vi "ProgressBar.vi"(9 "Bounds":T1, 11 "Settings":T4={"Name of test"="", "Date"=timestamp(0 s since 1904-01-01), "Location"="", "Template"="", "Soundcard"="", "resolution"=32, "Sampling rate"=48000, "Ch1 Gain "=25.0, "Ch2 Gain"=10.0, "Sample time (s)"=0.3, "Pre-trigger (s)"=0.01, "Hammer Threshold"=10.0, "Positions"=12, "Taps/Position"=5, "Set Names"="", "Freq resolution"=10.0, "Hammer cutoff"=0.0, "Mic cutoff"=0.0, "Double bounce "=0.0, "Hammer Cal"=10.0, "dB Offset"=0.0, "Accel Cal"=10.0, "Vibrometer Cal"=0.0, "Mic Cal"=0.0, "Output"=2, "Voltage Cal"=1.0, "Vibrometer Port"="ASRL27::INSTR", "Range"=4, "High Pass"=2, "Bandwidth"=4, "X Range"=[], "Y Range"=[], "dB Spread"=0.0, "Trigger"=0, "Ch_1"=25, "Ch_2"=25, "flip?"=FALSE, "60Hz"=FALSE, "Time offset"=0.0, "Piezo Cal"=1.0, "Default Notes"=""} {"Ch_2" min=1 step=1; "Ch_1" min=1 max=100 step=1; "Trigger" items=["Hammer (force)", "Self-tap", "Spacebar"]; "Bandwidth" items=["1 kHz"=1, "5 kHz"=5, "10 kHz"=10, "25 kHz"=25, "50 kHz"=50, "100 kHz"=100]; "High Pass" items=["Off", "13 Hz", "104 Hz"]; "Range" items=["10 mm/s"=1, "20 mm/s"=2, "50 mm/s"=5, "100 mm/s"=10, "200 mm/s"=20, "500 mm/s"=50, "1 m/s"=100, "2 m/s"=200]; "Output" items=["Accelerometer", "Speed (from acceleration)", "Microphone", "Vibrometer", "Piezo"]; "Voltage Cal" format="%#_13g"; "Ch2 Gain" format="%#_13g"; "Ch1 Gain" format="%#_13g"; "Double bounce" min=0.0; "Mic cutoff" min=0.0 format="%#_4g"; "Hammer cutoff" min=0.0 format="%#_4g"; "Freq resolution" min=0.0; "Pre-trigger (s)" format="%#_13g"; "Date" format="%<%H:%M\n%d/%m/%y>T"; "resolution" items=["16 bit"=16, "24 bit"=24, "32 bit"=32]; "Sampling rate" items=["22050 samp/s"=22050, "44100 samp/s"=44100, "48000 samp/s"=48000]}) -> (1 "files":string[](array[string]), 2 "positions":T2(array[cluster]), 3 "Progress Bar":picture)   [LabVIEW 2022 SP3]
uses:
  PreferencesControl.ctl
  <vilib>/Utility/miscctls.llb/LVBoundsTypeDef.ctl
panel:
  in  "Windows":T3={"Font Name:"="Times", "Size"=18, "Strikeout?"=FALSE, "Italic?"=FALSE, "Underline?"=FALSE, "Outline?"=FALSE, "Shadow?"=FALSE, "Bold?"=FALSE}
  out "Existing Data":string[](array[string])
  in  "Mac":T3={"Font Name:"="Times", "Size"=14, "Strikeout?"=FALSE, "Italic?"=FALSE, "Underline?"=FALSE, "Outline?"=FALSE, "Shadow?"=FALSE, "Bold?"=FALSE}
  # "Hz"
  # "dB"
  # "dB"
  # "sec"
  # "sec"
  # "mV/Pa"
  # "mV/m/s2"
  # "mV/mm/s"
  # "V/N"
  # "sec"
  # "sec"
  # "mV/N"
  # "a.u."
  # "a.u."
  # "sec"
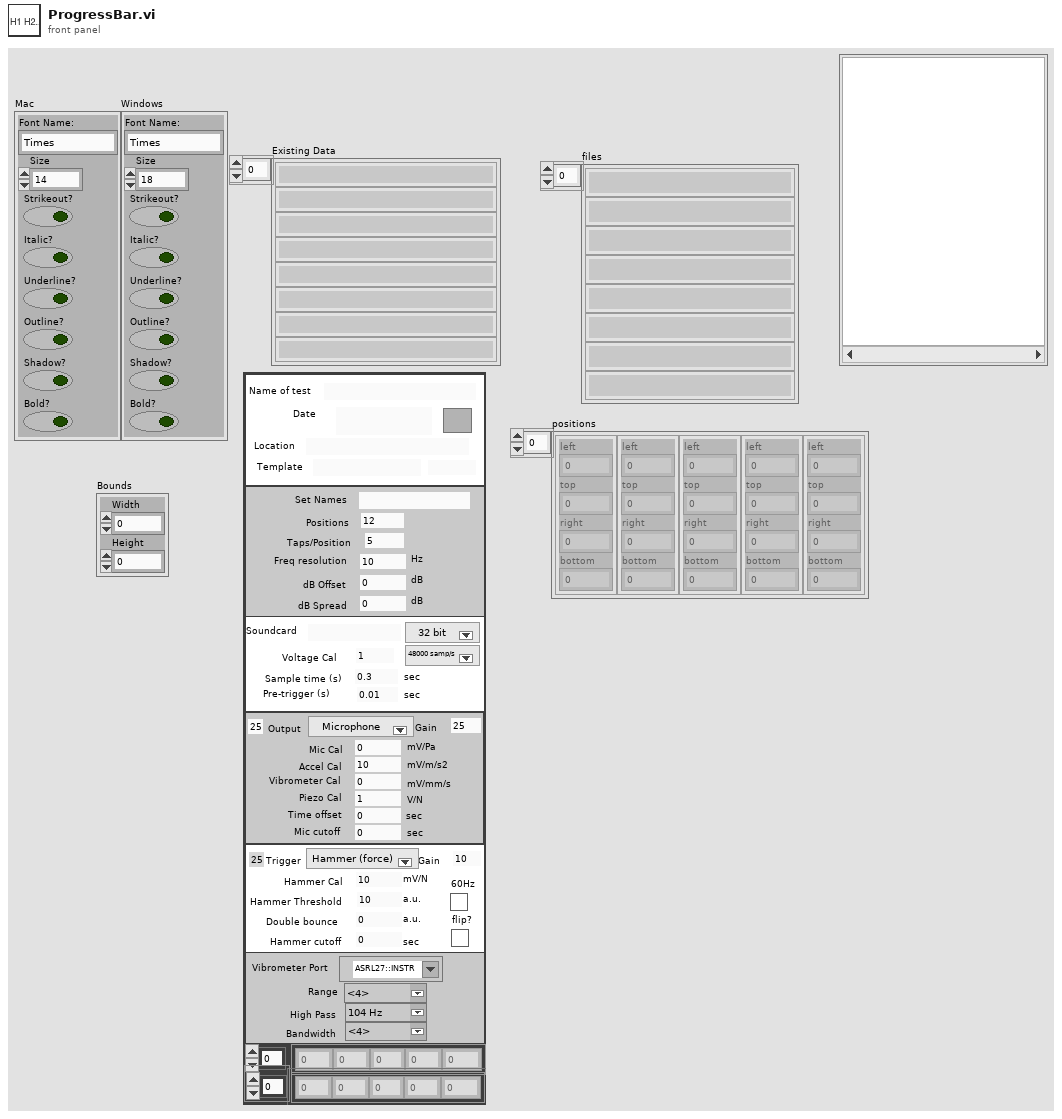
[diagram p1: front panel]
types:
  T1 = typedef "LVBoundsTypeDef.ctl" = cluster{"Width":u32, "Height":u32}
  T2 = cluster{"left":i16, "top":i16, "right":i16, "bottom":i16}[]
  T3 = cluster{"Font Name:":string, "Size":i16, "Strikeout?":bool, "Italic?":bool, "Underline?":bool, "Outline?":bool, "Shadow?":bool, "Bold?":bool}
  T4 = typedef "PreferencesControl.ctl" = cluster{"Name of test":string, "Date":timestamp, "Location":string, "Template":string, "Soundcard":string, "resolution":u16, "Sampling rate":u16, "Ch1 Gain ":dbl, "Ch2 Gain":dbl, "Sample time (s)":dbl, "Pre-trigger (s)":dbl, "Hammer Threshold":dbl, "Positions":i16, "Taps/Position":i16, "Set Names":string, "Freq resolution":dbl, "Hammer cutoff":dbl, "Mic cutoff":dbl, "Double bounce ":dbl, "Hammer Cal":dbl, "dB Offset":dbl, "Accel Cal":dbl, "Vibrometer Cal":dbl, "Mic Cal":dbl, "Output":u16, "Voltage Cal":dbl, "Vibrometer Port":refnum<visa-resource-name>, "Range":u16, "High Pass":u16, "Bandwidth":u16, "X Range":cluster{"Minimum":dbl, "Maximum":dbl, "Increment":dbl, "Minor Increment":dbl, "Start":dbl}[], "Y Range":cluster{"Minimum":dbl, "Maximum":dbl, "Increment":dbl, "Minor Increment":dbl, "Start":dbl}[], "dB Spread":dbl, "Trigger":u16, "Ch_1":u8, "Ch_2":u8, "flip?":bool, "60Hz":bool, "Time offset":dbl, "Piezo Cal":dbl, "Default Notes":string}
  T5 = enum16{"User-specified Font", "Application Font", "System Font", "Dialog Font"}
  T6 = cluster{"Width":i16, "Style":enum32{"Solid", "Dash", "Dot", "DashDot", "DashDotDot"}}
  T7 = cluster{"left":i16, "top":i16, "right":i16, "bottom":i16}
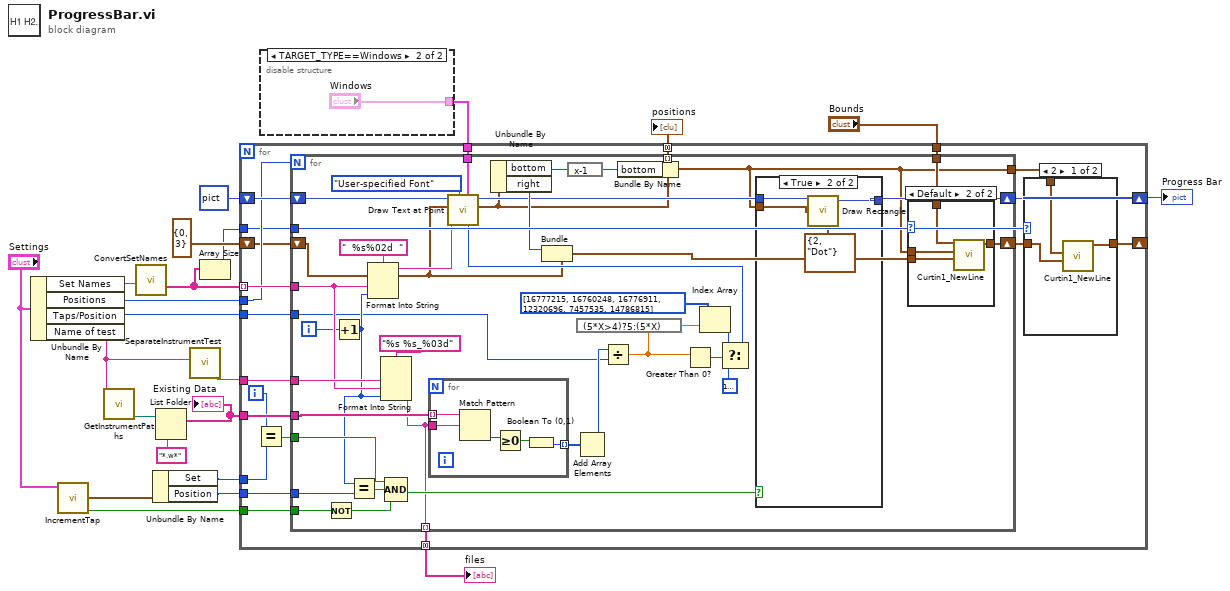
[diagram p0: block diagram]
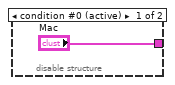
[diagram p2: hidden frame]
diagram:
  n1 = Unbundle By Name("Settings") -> ("Set Names"=w15:string, "Positions"=w14:i16, "Taps/Position"=w13:i16, "Name of test"=w5:string)
  n2 = call "IncrementTap.vi"("Settings"="Settings") -> ("Done?"=w9:bool, "Location"=w12:cluster{"Set":i16, "Position":i16, "Tap":i16})  [unwired: 5 in, 4 out]
  n3 = call "GetInstrumentPaths.vi"("Instrument"=w5) -> ("Path To Raw Folder"=w17:path)  [unwired: 6 in, 4 out]
  n4 = call "ConvertSetNames.vi"("Set Names"=w15) -> ("Set Names"=w2:string[])  [unwired: 10 in]
  n5 = Unbundle By Name(w12) -> ("Set"=w11:i16, "Position"=w10:i16)
  n6 = List Folder(path=w17, pattern="*.w*") -> (filenames=w18:string[])  [unwired: 2 in, 3 out]
  "Existing Data" <- w18
  n7 = call "SeparateInstrumentTest.vi"("Instrument"=w5) -> ("Just test"=w4:string)  [unwired: 6 in, 4 out]
  n8 = Array Size(array=w2) -> (size(s)=w1:i32)
  n9 = disable-structure shown="TARGET_TYPE==Windows" {
    disable-tunnel: ["Mac" "Windows"] -> w19
    frame condition #0 (active) {
    }
    frame condition #1 {
    }
  }
  n10 = for {
    tunnel: w2 -> [w45] mode=indexing
    tunnel: w14 -> [w42]
    shift-right: [w43] -> w21
    shift-left: picture data[5B] ("new picture") -> [w44]
    shift-right: [w27] -> _
    shift-left: cluster{"x":i16, "y":i16} {"x"=0, "y"=3} ("origin") -> [w41]
    tunnel: w19 -> [w40]
    tunnel: w4 -> [w39]
    tunnel: w18 -> [w38]
    tunnel: w13 -> [w37]
    tunnel: w11 -> [w35]
    tunnel: w10 -> [w34]
    tunnel: w9 -> [w32]
    tunnel: [w31] -> w7 mode=concatenating
    tunnel: [w30] -> w6 mode=concatenating
    tunnel: "Bounds" -> [w29]
    tunnel: w1 -> [w28]
    i -> [w36]
    n11 = Equal?(x=w36, y=w35) -> (x = y?=w33:bool)
    n12 = for {
      N: w42 -> [_]
      tunnel: w45 -> [w73]
      shift-right: [w67] -> w43
      shift-left: w44 -> [w88]
      shift-right: [w53] -> w26
      shift-left: w41 -> [w57]
      tunnel: w40 -> [w86]
      tunnel: w39 -> [w83]
      tunnel: w38 -> [w82]
      tunnel: w37 -> [w55]
      tunnel: w34 -> [w71]
      tunnel: w33 -> [w69]
      tunnel: w32 -> [w65]
      tunnel: [w60] -> w31 mode=indexing
      tunnel: [w58] -> w30 mode=indexing
      tunnel: w29 -> [w52]
      tunnel: w28 -> [w51]
      tunnel: [w50] -> w25
      i -> [w72]
      n13 = Not(x=w65) -> (.not. x?=w64:bool)
      n14 = Increment(x=w72) -> (x+1=w63:i32)
      n15 = Equal?(x=w63, y=w71) -> (x = y?=w70:bool)
      n16 = Format Into String(format string="  %s%02d  ", w73, w63) -> (resulting string=w59:string)  [unwired: 2 in, 1 out]
      n17 = Format Into String(format string="%s %s_%03d", w83, w73, w63) -> (resulting string=w58:string)  [unwired: 2 in, 1 out]
      n18 = Compound Arithmetic op=AND(w69, w70, w64) -> (w66:bool)
      n19 = for {
        tunnel: w82 -> [w104] mode=indexing
        tunnel: w58 -> [w103]
        tunnel: [w100] -> w81 mode=indexing
        n20 = Match Pattern(string=w104, regular expression=w103) -> (offset past match=w102:i32)  [unwired: 1 in, 3 out]
        n21 = Greater Or Equal To 0?(x=w102) -> (x >= 0?=w101:bool)
        n22 = Boolean To (0,1)(Boolean=w101) -> (0, 1=w100:i16)
      }
      n23 = Add Array Elements(numeric array=w81) -> (sum=w56:i16)
      n24 = Divide(x=w56, y=w55) -> (x/y=w75:dbl)
      n25 = expression code="(5*X>4)?5:(5*X)"(w75) -> (w74:dbl)
      n26 = Greater Than 0?(x=w75) -> (x > 0?=w80:bool)
      n27 = Index Array(array=u32[] [16777215, 16760248, 16776911, 12320696, 7457535, 14786815], index=w74) -> (element=w76:u32)
      n28 = Select(t=w76, s=w80, f=u32 16777216 ("BG color(transparent)")) -> (s? t:f=w78:u32)
      n29 = call <vilib>:"Draw Text at Point.vi"("BG color(transparent)"=w78, "[user-specified font]"=w86, "desired font(Application)"=T5."User-specified Font", "text"=w59, "origin"=w57, "picture"=w88) -> ("text rect"=w60:T7, "new picture"=w68:picture)  [unwired: 4 in]
      n30 = Unbundle By Name(w60) -> ("bottom"=w62:i16, "right"=w87:i16)
      n31 = Bundle(cluster=w57, "x"=w87) -> (w54:cluster{"x":i16, "y":i16})  [unwired: 1 in]
      n32 = expression code="x-1"(w62) -> (w61:i16)
      n33 = Bundle By Name(cluster=w60, "bottom"=w61) -> (w50:T7)
      n34 = case shown="True" w66 {
        tunnel: w68 -> [w95 w99]
        tunnel: w50 -> [_ w96]
        tunnel: [w95 w98] -> w67
        frame False {
        }
        frame True {
          n35 = call <vilib>:"Draw Rectangle.vi"("picture"=w99, "rect"=w96, "pen"=T6 {"Width"=2, "Style"=enum."Dot"}) -> ("new picture"=w98:picture)  [unwired: 6 in]
        }
      }
      n36 = case shown="Default" w51 {
        tunnel: w54 -> [w90 w94]
        tunnel: [w90 w93] -> w53
        tunnel: w50 -> [_ w92]
        tunnel: w52 -> [_ w91]
        frame 2 {
        }
        frame Default {
          n37 = call "Curtin1_NewLine.vi"("origin in"=w94, "text rect"=w92, "Bounds"=w91) -> ("origin out"=w93:cluster{"x":i16, "y":i16})  [unwired: 8 in]
        }
      }
    }
    n38 = case shown="2" w28 {
      tunnel: [w48 w49] -> w27
      tunnel: w26 -> [w47 w49]
      tunnel: w25 -> [w46 _]
      frame 2 {
        n39 = call "Curtin1_NewLine.vi"("origin in"=w47, "text rect"=w46) -> ("origin out"=w48:cluster{"x":i16, "y":i16})  [unwired: 9 in]
      }
      frame Default {
      }
    }
  }
  "Progress Bar" <- w21
  "positions" <- w7
  "files" <- w6
